vi "num2str.vi"(11 "NumArray":i32[](array[numeric])) -> (3 "StrArray":string[](array[string]))   [LabVIEW 2018, in "AcPwrPlugins.lvlib" / "NHRGridSim.lvclass"]
doc: "Converts an array that has a pair of numeric values into a similar array that has the string representation of those numeric values."
uses:
  NHRGridSim.lvclass
panel:
  # "This VI takes a pair of integer values that is passed as an array of two elements, and creates an equivalent array for the string representation of those values. Like:\n                   [ 5, 20 ]   --->    [ \"5\", \"20\" ]\n\n  It's mostly to have a very small VI icon for this task."
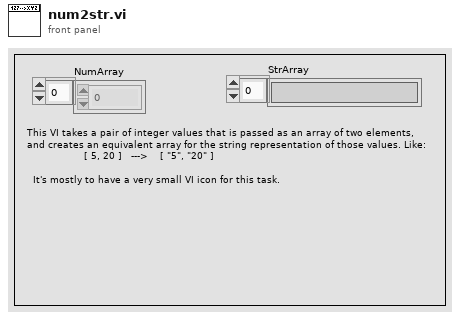
[diagram p1: front panel]
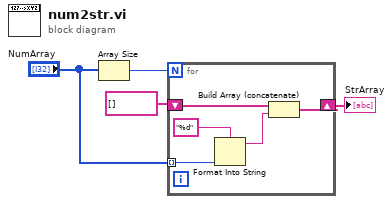
[diagram p0: block diagram]
diagram:
  n1 = Array Size(array="NumArray") -> (size(s)=w4:i32)
  n2 = for {
    N: w4 -> [_]
    tunnel: "NumArray" -> [w9] mode=indexing
    shift-right: [w7] -> w1
    shift-left: string[] [] -> [w5]
    n3 = Format Into String(format string="%d", w9) -> (resulting string=w6:string)  [unwired: 2 in, 1 out]
    n4 = Build Array (concatenate)(w5, w6) -> (w7:string[])
  }
  "StrArray" <- w1
